vi "Action Engine.vi"() -> ()   [LabVIEW 2021]
uses:
  controls/Timer State.ctl
panel:
  out "Master Out":bool
  out "Trigger":bool
  out "Clock Output":bool
  in  "Enum":T1=enum."Start Timer"
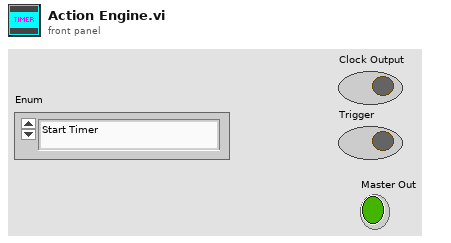
[diagram p1: front panel]
types:
  T1 = typedef "Timer State.ctl" = enum16{"Check Timer", "Start Timer", "Pause Timer", "Exit Timer"}
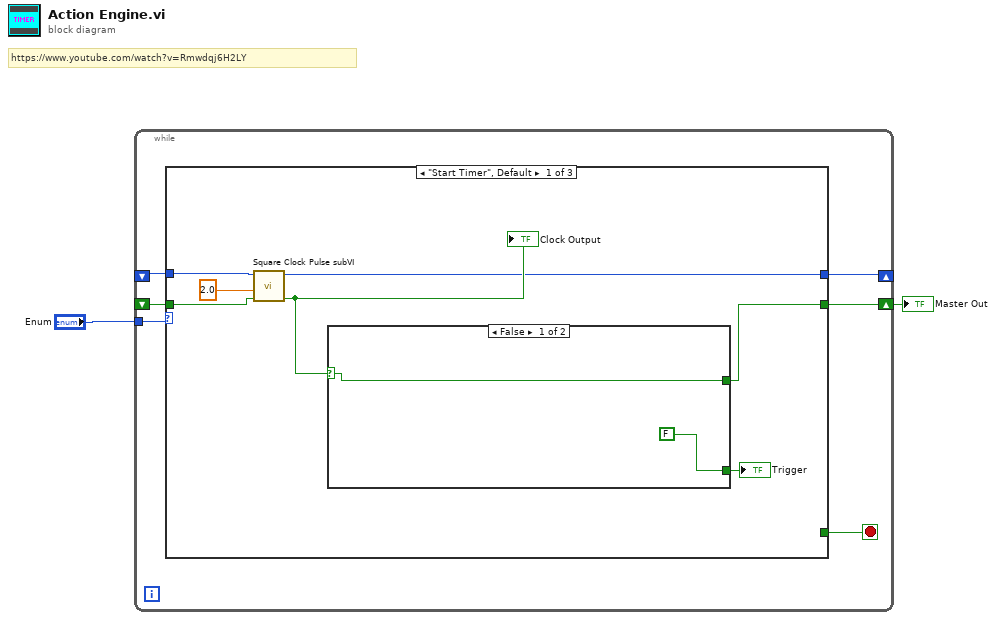
[diagram p0: block diagram]
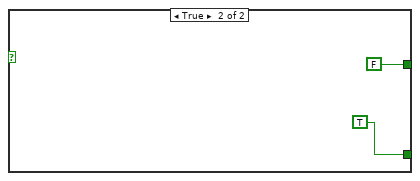
[diagram p2: hidden frame]
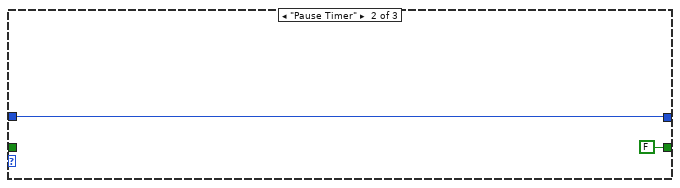
[diagram p3: hidden frame]
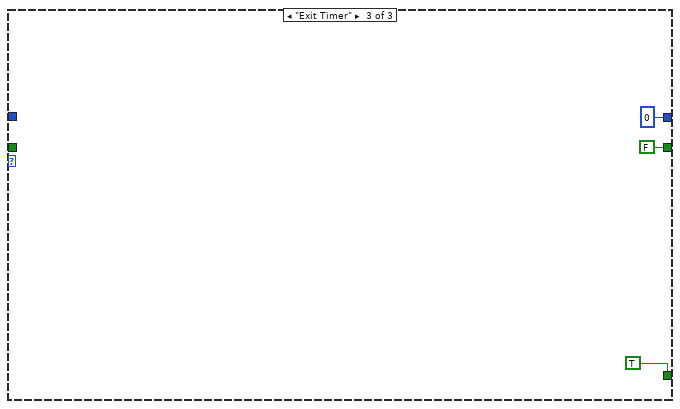
[diagram p4: hidden frame]
diagram:
  # "https://www.youtube.com/watch?v=Rmwdqj6H2LY"
  n1 = while {
    tunnel: "Enum" -> [w8]
    shift-right: [w7] -> _
    shift-left: _ -> [w6]
    shift-right: [w5] -> w1
    shift-left: _ -> [w4]
    stop <- w3 stop-if-true
    n2 = case shown="\"Start Timer\", Default" w8 {
      tunnel: [w13 w20 u32 0 ("Last Event mS")] -> w7
      tunnel: w6 -> [w12 w20 _]
      tunnel: [w11 FALSE ("Clock Output") FALSE ("Clock Output")] -> w5
      tunnel: w4 -> [w10 _ _]
      tunnel: [_ _ TRUE] -> w3
      frame "Start Timer", Default {
        n3 = call "Square Clock Pulse subVI.vi"("Last Bool State"=w10, "Sample Rate (Hz)"=2.0, "Last Event mS"=w12) -> ("Clock Output"=w14:bool, "Last Event mS"=w13:u32)  [unwired: 5 in, 2 out]
        "Clock Output" <- w14
        n4 = case shown="False" w14 {
          selector: w14 -> [w17 _]
          tunnel: [w17 FALSE ("Clock Output")] -> w11
          tunnel: [FALSE ("Trigger") TRUE ("Trigger")] -> w9
          frame False {
          }
          frame True {
          }
        }
        "Trigger" <- w9
      }
      frame "Pause Timer" {
      }
      frame "Exit Timer" {
      }
    }
  }
  "Master Out" <- w1
